vi "phase diff tester.vi"() -> ()   [LabVIEW 2021]
uses:
  <instrlib>/_niInstr/DSP/v1/Shared/Public/IQ Data.ctl
  <instrlib>/_niInstr/DSP/v1/FPGA/Public/Sub VIs/Frequency Shift/Frequency Shift - 1 spc.vi
  <instrlib>/_niInstr/DSP/v1/FPGA/niInstr DSP v1 FPGA.lvlib
  <instrlib>/_niInstr/DSP/v1/Shared/niInstr DSP v1 Shared.lvlib
panel:
  in  "phase":fxp<+/-,21,0>
  out "Waveform Chart":dbl[][](graph)
  out "Waveform Graph":cluster{"f0":dbl, "df":dbl, "magnitude":dbl[]}[](graph)
  in  "number of sampels":dbl
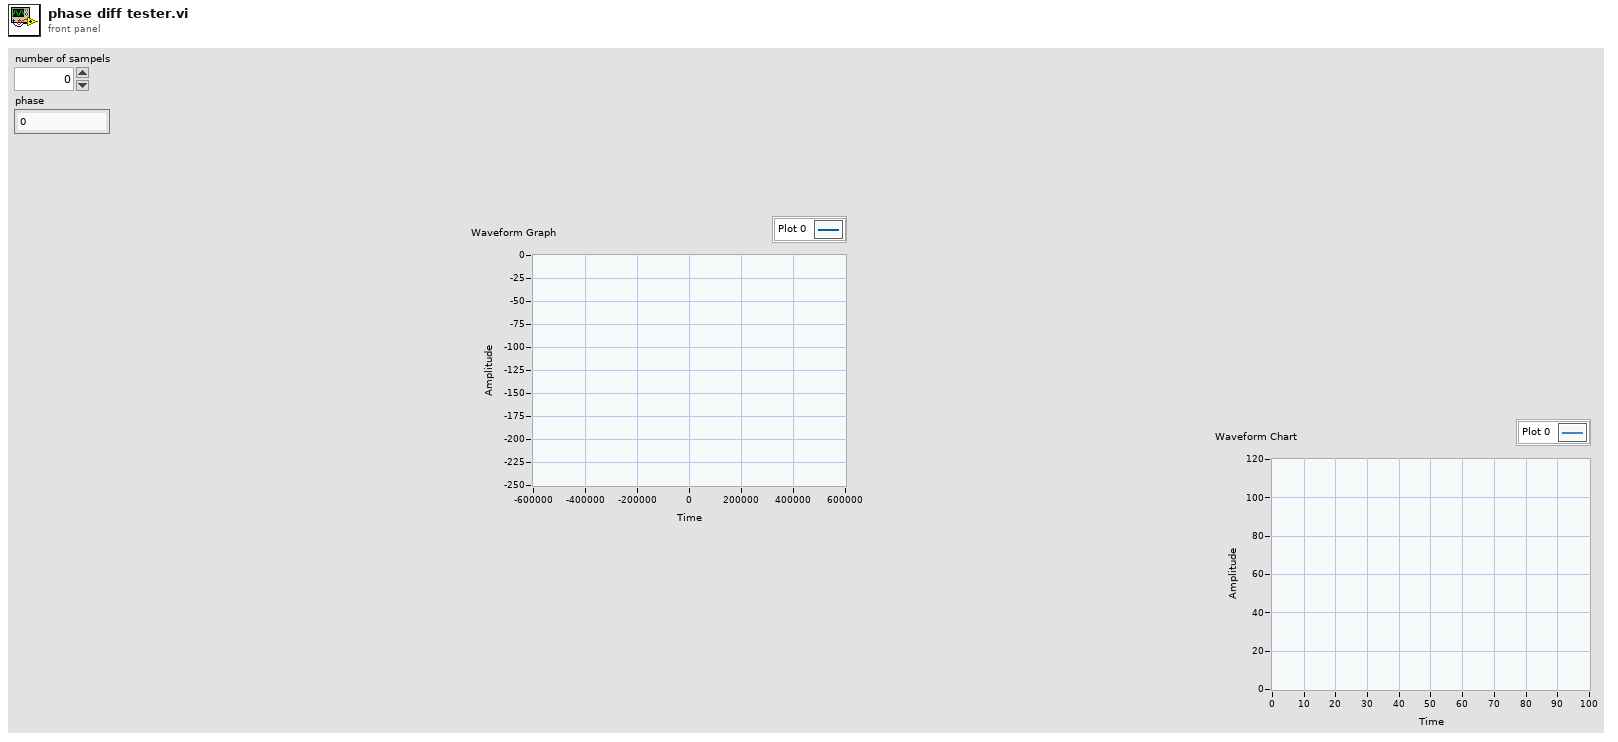
[diagram p1: front panel]
types:
  T1 = typedef "niInstr DSP v1 Shared.lvlib/IQ Data.ctl" = cluster{"I":fxp<+/-,18,1>, "Q":fxp<+/-,18,1>, "overflow":bool}
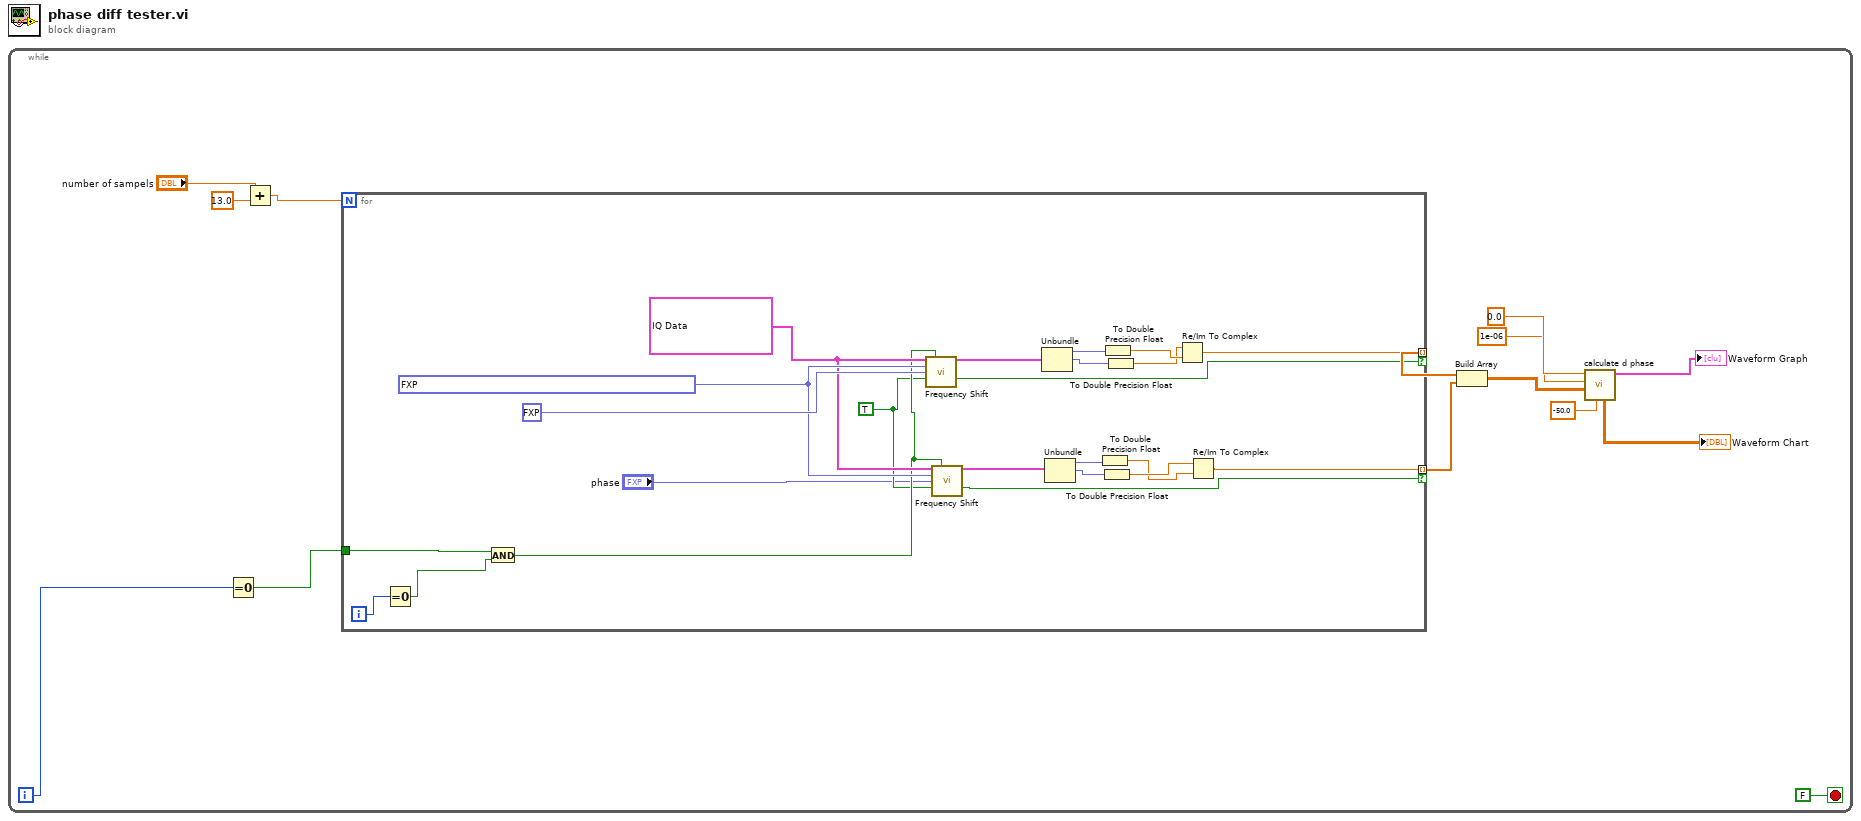
[diagram p0: block diagram]
diagram:
  n1 = while {
    i -> [w2]
    stop <- FALSE stop-if-true
    n2 = Equal To 0?(x=w2) -> (x = 0?=w1:bool)
    n3 = Add(x="number of sampels", y=13.0) -> (x+y=w14:dbl)
    n4 = for {
      N: w14 -> [_]
      tunnel: [w24] -> w10 mode=indexing if=w22
      tunnel: [w23] -> w11 mode=indexing if=w21
      tunnel: w1 -> [w20]
      i -> [w19]
      w16 = TRUE ("input valid")
      w35 = T1 {"I"=0.09999847412109375, "Q"=0.0, "overflow"=FALSE} ("data")
      w36 = fxp<+/-,48,0> 0.10000000000000142 ("frequency shift")
      n5 = Equal To 0?(x=w19) -> (x = 0?=w18:bool)
      n6 = And(x=w20, y=w18) -> (x .and. y?=w17:bool)
      n7 = call-poly <instrlib>:"Frequency Shift.vi"("data in"=w35, "reset"=w17, "frequency shift"=w36, "phase"=fxp<+/-,21,0> 0.0, "input valid"=w16) -> ("data out"=w34:T1, "output valid"=w21:bool)  [unwired: 7 in, 2 out]
      n8 = call-poly <instrlib>:"Frequency Shift.vi"("data in"=w35, "reset"=w17, "frequency shift"=w36, "phase"="phase", "input valid"=w16) -> ("data out"=w33:T1, "output valid"=w22:bool)  [unwired: 7 in, 2 out]
      n9 = Unbundle(w34) -> ("I"=w32:fxp<+/-,18,1>, "Q"=w31:fxp<+/-,18,1>)  [unwired: 1 out]
      n10 = Unbundle(w33) -> ("I"=w30:fxp<+/-,18,1>, "Q"=w29:fxp<+/-,18,1>)  [unwired: 1 out]
      n11 = To Double Precision Float(number=w30) -> (double precision float=w25:dbl)
      n12 = To Double Precision Float(number=w29) -> (double precision float=w26:dbl)
      n13 = To Double Precision Float(number=w32) -> (double precision float=w28:dbl)
      n14 = To Double Precision Float(number=w31) -> (double precision float=w27:dbl)
      n15 = Re/Im To Complex(1:w28, 2:w27) -> (0:w23:cdb)
      n16 = Re/Im To Complex(1:w25, 2:w26) -> (0:w24:cdb)
    }
    n17 = Build Array(w11, w10) -> (w7:cdb[][])
    n18 = call "calculate d phase.vi"("threshold"=-50.0, "IQ in"=w7, "dt"=1e-06, "center frequency (Hz)"=0.0) -> ("spectrum"=→"Waveform Graph":cluster{"f0":dbl, "df":dbl, "magnitude":dbl[]}[], "d phase"=→"Waveform Chart":dbl[][])  [unwired: 3 in, 3 out]
  }
